vi "Read Write Name.vi"(7 "Read(f)\nWrite(t)":T1, 10 "Name":string, 11 "WavBuf":refnum<class "WavBuf.lvclass">) -> (2 "Name Out":string, 3 "WavBuf Out":refnum<class "WavBuf.lvclass">)   [LabVIEW 2020, in "WavBuf.lvclass"]
uses:
  WavBuf.lvclass
  Universal Controls/Read Write Button.ctl
  WavBuf.lvclass/WavBuf.ctl
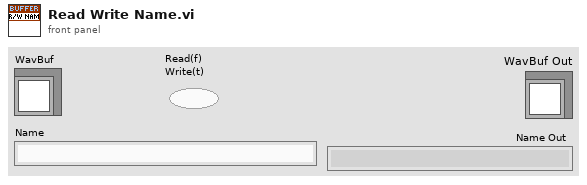
[diagram p1: front panel]
types:
  T1 = typedef "Read Write Button.ctl" = bool
  T2 = typedef "Ref_DVR_Buffer.ctl" = refnum<data-value>
  T3 = typedef "Waveform_Data.ctl" = waveform(dbl)
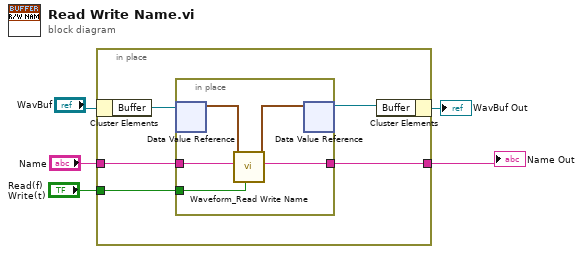
[diagram p0: block diagram]
diagram:
  n1 = in-place {
    in-place-border: [w10] -> w5
    in-place-border: "Name" -> [w9]
    in-place-border: "Read(f)\nWrite(t)" -> [w8]
    n2 = in-place-cluster #1("WavBuf") -> ("Buffer"=w7:T2)
    n3 = in-place {
      in-place-border: [w15] -> w10
      in-place-border: w9 -> [w14]
      in-place-border: w8 -> [w13]
      n4 = in-place-dvr #2(w7) -> (w12:T3)  [unwired: 1 out]
      n5 = call "Waveform_Read Write Name.vi"("Read(f)\nWrite(t)"=w13, "Name"=w14, "Raw Data Waveform"=w12) -> ("Name Out"=w15:string, "Raw Data Waveform Out"=w11:T3)  [unwired: 7 in]
      n6 = in-place-dvr #2(w11) -> (w6:T2)  [unwired: 1 out]
    }
    n7 = in-place-cluster #1("Buffer"=w6) -> (→"WavBuf Out":refnum<class "WavBuf.lvclass">)
  }
  "Name Out" <- w5
